vi "Subscribe.vi"(8 "error in (no error)":errorcluster, 10 "Subscription Request":refnum<class "SubscriptionRequest.lvclass">, 11 "Mediator In":refnum<class "Mediator.lvclass">) -> (0 "error out":errorcluster, 3 "Mediator Out":refnum<class "Mediator.lvclass">)   [LabVIEW 2017, in "Mediator.lvlib" / "Mediator.lvclass"]
doc: "<License>\nCopyright © 2017 Composed Systems, LLC | All rights reserved\nwww.composed.io\n\nAuthor: Ethan Stern <ethan.stern@composed.io>\n\nThis software is provided \"AS IS\" WITHOUT WARRANTIES, either express or implied, AND IS FOR EDUCATIONAL PURPOSES ONLY.\n</License>"
uses:
  Mediator.lvclass
  IMediator/SubscriptionRequest/SubscriptionRequest.lvclass
  Mediator.lvclass/Mediator.ctl
  IMediator/SubscriptionRequest/SubscriptionRequest.lvclass/SubscriptionRequest.ctl
  TopicLookupTable/TopicLookupTable.lvclass/TopicLookupTable.ctl
  Topic Messages/Add Topic Subscriber Msg/Add Topic Subscriber Msg.lvclass/Add Topic Subscriber Msg.ctl
  <vilib>/ActorFramework/Message Enqueuer/Message Enqueuer.lvclass/Message Enqueuer.ctl
  <vilib>/ActorFramework/Message Enqueuer/Enqueue.vi
  Topic Messages/Add Topic Subscriber Msg/Add Topic Subscriber Msg.lvclass
  C:/Program Files (x86)/National Instruments/LabVIEW 2017/vi.lib/ActorFramework/Message/Message.lvclass
  gpm_packages/@cs/variant/Source/Format Type String.vi
  <vilib>/ActorFramework/Message Priority Queue/Priority Enqueue.vi
  <vilib>/ActorFramework/Message Enqueuer/Message Enqueuer.lvclass
  TopicLookupTable/TopicLookupTable.lvclass
panel:
  # "What does subscriber want? (Datum Name and Type)\nHow does it get sent? (Transport)\nUnder what conditions? (SubscriptionPolicy)"
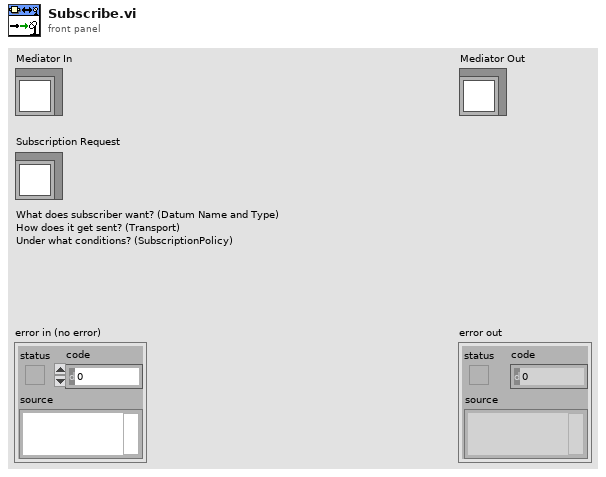
[diagram p1: front panel]
types:
  T1 = typedef "IMediator.lvlib/ISubscriptionPolicy.lvclass/ISubscriptionPolicy Reference.ctl" = refnum<data-value>
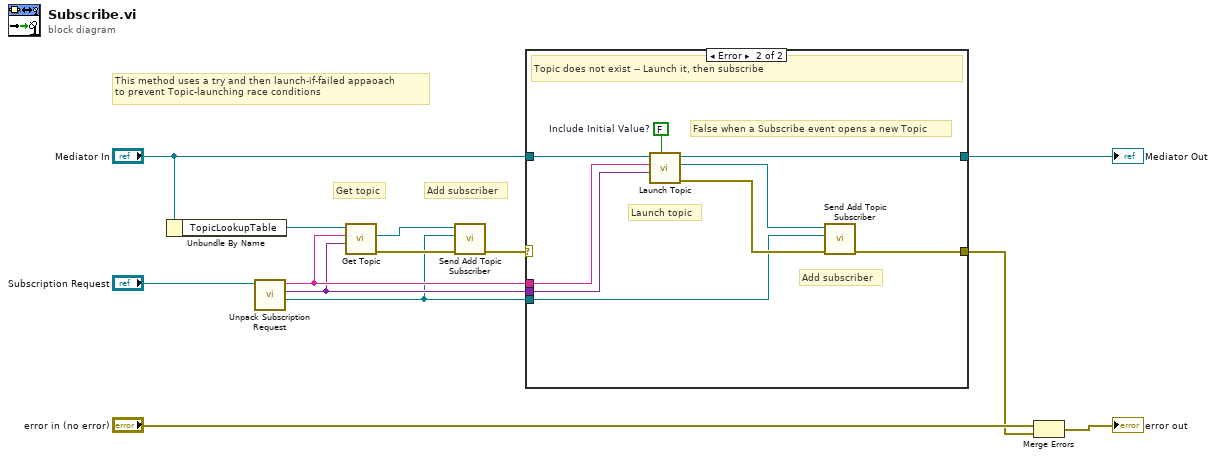
[diagram p0: block diagram]
diagram:
  # "This method uses a try and then launch-if-failed appaoach\nto prevent Topic-launching race conditions"
  # "Add subscriber"
  # "Get topic"
  n1 = Unbundle By Name("Mediator In") -> ("TopicLookupTable"=w3:refnum<data-value>)
  n2 = call "Unpack Subscription Request.vi"("SubscriptionRequest"="Subscription Request") -> ("Subscription Policy"=w2:T1, "Type"=w5:variant, "Datum Name"=w6:string)  [unwired: 8 in]
  n3 = call "Get Topic.vi"("Topic Type"=w5, "Topic Name"=w6, "TopicLookupTable"=w3) -> ("error out"=w7:errorcluster, "Topic Enqueuer"=w11:refnum<class "Message Enqueuer.lvclass">)  [unwired: 6 in, 1 out]
  n4 = call "Send Add Topic Subscriber.vi"("error in (no error)"=w7, "Subscription Policy"=w2, "Message Enqueuer"=w11) -> ("error out"=w9:errorcluster)  [unwired: 7 in, 1 out]
  n5 = case shown="Error" w9 {
    selector: w9 -> [w14 _]
    tunnel: "Mediator In" -> [w15 w20]
    tunnel: [w15 w16] -> w1
    tunnel: w6 -> [_ w19]
    tunnel: w5 -> [_ w18]
    tunnel: [w14 w24] -> w8
    tunnel: w2 -> [_ w21]
    frame No Error {
      # "Topic exists -- Subscribe OK"
    }
    frame Error {
      w17 = FALSE  # Include Initial Value?
      # "False when a Subscribe event opens a new Topic"
      # "Launch topic"
      # "Add subscriber"
      # "Topic does not exist -- Launch it, then subscribe"
      n6 = call-dynamic "Launch Topic.vi"("Include Initial Value? (F)"=w17, "Type"=w18, "Datum Name"=w19, "Mediator in"=w20) -> ("error out"=w22:errorcluster, "New Topic Enqueuer"=w23:refnum<class "Message Enqueuer.lvclass">, "Mediator out"=w16:refnum<class "Mediator.lvclass">)  [unwired: 5 in]
      n7 = call "Send Add Topic Subscriber.vi"("error in (no error)"=w22, "Subscription Policy"=w21, "Message Enqueuer"=w23) -> ("error out"=w24:errorcluster)  [unwired: 7 in, 1 out]
    }
  }
  "Mediator Out" <- w1
  n8 = Merge Errors("error in (no error)", w8) -> (→"error out":errorcluster)
